vi "Test Cross Hierarchy.vi"() -> ()   [LabVIEW 2020]
uses:
  TSnax/Engine/Engine.lvclass
panel:
  out "VersionString":string
  out "error out":errorcluster
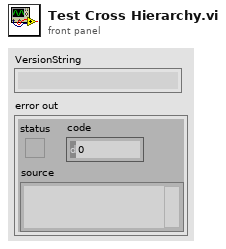
[diagram p1: front panel]
types:
  T1 = enum32{"Bad", "Idle", "Run top level", "Running"}
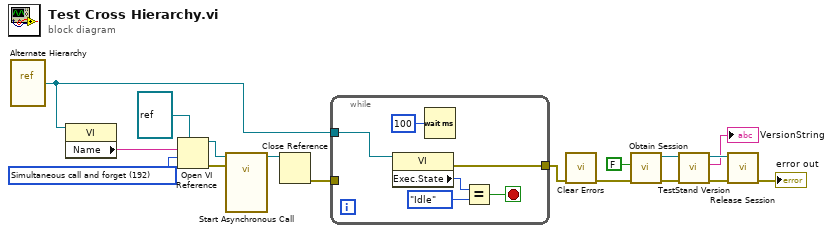
[diagram p0: block diagram]
diagram:
  w15 = 192 items=["Record modifications"=1, "Open templates for editing"=2, "Prompt user to save"=4, "Prepare for reentrant run"=8, "Prompt to find missing subVIs"=16, "Hide loading dialog box"=32, "Enable simultaneous calls"=64, "Prepare to call and forget"=128, "Simultaneous call and forget"=192, "Prepare to call and collect"=256, "Simultaneous call and collect"=320]
  n1 = vi-ref "Alternate Hierarchy.vi"() -> (w4:refnum<vi>)
  n2 = property class="VI"(reference=w4) -> ("Name"=w14:string)  [unwired: 1 in, 2 out]
  n3 = Open VI Reference(type specifier VI Refnum (for type only)=refnum<vi> refnum, vi path=w14, options=w15) -> (vi reference=w17:refnum<vi>, error out=w16:errorcluster)  [unwired: 3 in]
  n4 = call-by-ref "Start Asynchronous Call"(reference=w17, error in=w16) -> (reference out=w3:refnum<vi>)  [unwired: 12 in, 1 out]
  n5 = Close Reference(reference=w3) -> (error out=w2:errorcluster)  [unwired: 1 in]
  n6 = while {
    tunnel: w4 -> [w22]
    tunnel: w2 -> [_]
    tunnel: [w21] -> w1
    stop <- w18 stop-if-true
    n7 = property class="VI"(reference=w22) -> (error out=w21:errorcluster, "Exec.State"=w20:T1)  [unwired: 1 in, 1 out]
    n8 = Wait (ms)(milliseconds to wait=u32 100) -> ()  [unwired: 1 out]
    n9 = Equal?(x=w20, y=T1."Idle") -> (x = y?=w18:bool)
  }
  n10 = call <vilib>:"Clear Errors.vi"("error in (no error)"=w1) -> ("error out"=w13:errorcluster)  [unwired: 5 in, 1 out]
  n11 = call "Obtain Session.vi"("error in (no error)"=w13, "Create if needed? (T)"=FALSE) -> ("error out"=w9:errorcluster, "Engine out"=w10:refnum<class "Engine.lvclass">)  [unwired: 8 in]
  n12 = call "TestStand Version.vi"("error in (no error)"=w9, "Engine in"=w10) -> ("error out"=w8:errorcluster, "VersionString"=→"VersionString":string, "Engine out"=w7:refnum<class "Engine.lvclass">)  [unwired: 7 in]
  n13 = call "Release Session.vi"("error in (no error)"=w8, "Engine in"=w7) -> ("error out"=→"error out":errorcluster)  [unwired: 9 in]
